vi "Result_Test.vi"(8 "error in (no error)":errorcluster caption="entrée d'erreur (pas d'erreur)", 11 "Flash_Jlink en entrée":refnum<class "Flash_SIN_Test_FW.lvclass">) -> (0 "error out":errorcluster caption="sortie d'erreur", 3 "Flash_Jlink en sortie":refnum<class "Flash_SIN_Test_FW.lvclass">)   [LabVIEW 2020, in "Library Test.lvlib" / "Flash_SIN_Test_FW.lvclass"]
uses:
  Flash_SIN_Test_FW.lvclass
  C:/Users/ngarcin/OneDrive - Altyor/Standard TB/Class/Test/Test (Default)/Test (Default).lvclass
  Flash_Commander/Flash_Commander.lvclass
  Flash_SIN_Test_FW.lvclass/Flash_SIN_Test_FW.ctl
panel:
  out "Ok":bool
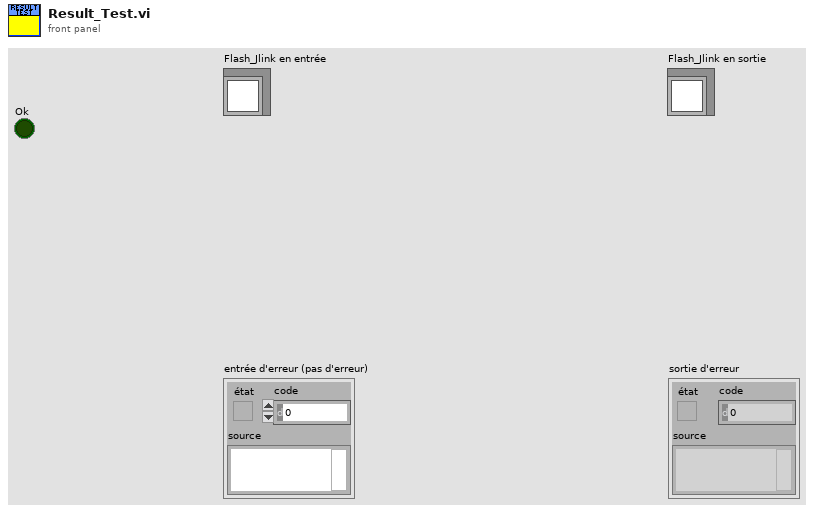
[diagram p1: front panel]
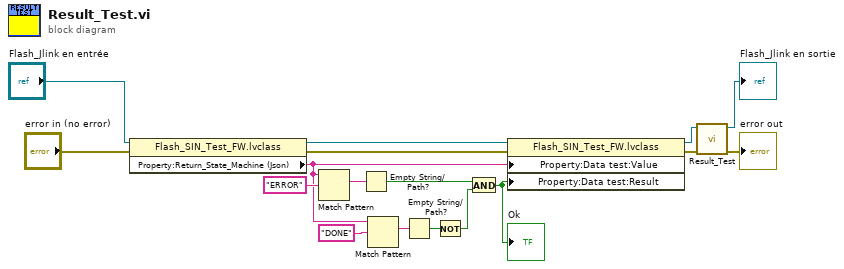
[diagram p0: block diagram]
diagram:
  n1 = property class="Flash_SIN_Test_FW.lvclass"(reference="Flash_Jlink en entrée", error in="error in (no error)") -> (reference out=w12:refnum<class "Flash_SIN_Test_FW.lvclass">, error out=w13:errorcluster, "Property:Return_State_Machine (Json)"=w7:string)
  n2 = Match Pattern(string=w7, regular expression="ERROR" ("expression régulière")) -> (match substring=w15:string)  [unwired: 1 in, 3 out]
  n3 = Empty String/Path?(string/path=w15) -> (empty?=w9:bool)
  n4 = Match Pattern(string=w7, regular expression="DONE" ("expression régulière")) -> (match substring=w11:string)  [unwired: 1 in, 3 out]
  n5 = Empty String/Path?(string/path=w11) -> (empty?=w10:bool)
  n6 = Not(x=w10) -> (.not. x?=w6:bool)
  n7 = And(x=w9, y=w6) -> (x .and. y?=w8:bool)
  "Ok" <- w8
  n8 = property class="Flash_SIN_Test_FW.lvclass"(reference=w12, error in=w13, "Property:Data test:Value"=w7, "Property:Data test:Result"=w8) -> (reference out=w1:refnum<class "Flash_SIN_Test_FW.lvclass">, error out=w2:errorcluster)
  n9 = call-parent "Result_Test.vi"("error in (no error)"=w2, "Flash_Jlink en entrée"=w1) -> ("error out"=→"error out":errorcluster, "Flash_Jlink en sortie"=→"Flash_Jlink en sortie":refnum<class "Flash_SIN_Test_FW.lvclass">)  [unwired: 8 in]
